vi "Init P2P stream.vi"(7 "single shot":bool, 8 "Trigger ource":T1, 9 "input impedance":u32(ring) caption="Input Impedance" items=["1 mega ohm"=0, "50 ohms"=2], 10 "SCOPE Resource":refnum<k15>="Dev1" caption="NI-Scope Resource", 11 "FPGA VI Reference":T3) -> (0 "error out":errorcluster, 2 "P2P params":T2={"instrument handle"="", "stream session"=refnum, "scale"={"offset"=0.0, "gain"=0.0, "reserved 1"=0.0, "reserved 2"=0.0}, "actual sample rate"=10000000.0, "Trigger"=enum."PFI 0", "SCOPE Resource"="Dev1", "input impedance"=0} {"input impedance" items=["1 mega ohm"=0, "50 ohms"=2]; "actual sample rate" format="%.2p"}, 3 "FPGA VI Reference out":T3)   [LabVIEW 2013]
uses:
  Config/5160FPGAref.ctl
  P2P params.ctl
  trigger_source.ctl
  <instrlib>/niScope/Controls/niScope vertical coupling.ctl
  <instrlib>/niScope/Controls/niScope trigger slope.ctl
  <instrlib>/niScope/Controls/niScope trigger source digital.ctl
  <instrlib>/niScope/Acquire/niScope Get Scaling Coefficients.vi
  <vilib>/FPGAPlugInAG/Dynamic/niLvFpga_P2PGetEndpoint_Dynamic.vi
  <instrlib>/niScope/Configure/Trigger/niScope Configure Trigger Software.vi
  <instrlib>/niScope/Configure/Trigger/niScope Configure Trigger Digital.vi
  <vilib>/rvi/interface/nirviMethod/nirviMethod.xnode
  <vilib>/rvi/errors/niLvFpgaMergeErrorWithErrorCode.vi
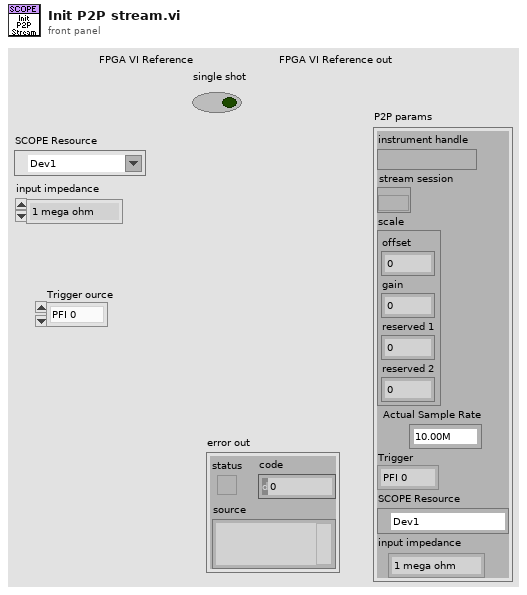
[diagram p1: front panel]
types:
  T1 = typedef "trigger_source.ctl" = enum16{"PFI 0", "PFI 1", "Software"}
  T2 = typedef "P2P params.ctl" = cluster{"instrument handle":refnum<k15>, "stream session":refnum<k20>, "scale":cluster{"offset":dbl, "gain":dbl, "reserved 1":dbl, "reserved 2":dbl}, "actual sample rate":dbl, "Trigger":T1, "SCOPE Resource":refnum<k15>, "input impedance":u32}
  T3 = typedef "5160FPGAref.ctl" = refnum<k20>
  T4 = typedef "niScope vertical coupling.ctl" = i32
  T5 = cluster{"offset":dbl, "gain":dbl, "reserved 1":dbl, "reserved 2":dbl}[]
  T6 = cluster{"coefficient info[0]":cluster{"offset":dbl, "gain":dbl, "reserved 1":dbl, "reserved 2":dbl}, "coefficient info[1]":cluster{"offset":dbl, "gain":dbl, "reserved 1":dbl, "reserved 2":dbl}, "coefficient info[2]":cluster{"offset":dbl, "gain":dbl, "reserved 1":dbl, "reserved 2":dbl}, "coefficient info[3]":cluster{"offset":dbl, "gain":dbl, "reserved 1":dbl, "reserved 2":dbl}, "coefficient info[4]":cluster{"offset":dbl, "gain":dbl, "reserved 1":dbl, "reserved 2":dbl}, "coefficient info[5]":cluster{"offset":dbl, "gain":dbl, "reserved 1":dbl, "reserved 2":dbl}, "coefficient info[6]":cluster{"offset":dbl, "gain":dbl, "reserved 1":dbl, "reserved 2":dbl}, "coefficient info[7]":cluster{"offset":dbl, "gain":dbl, "reserved 1":dbl, "reserved 2":dbl}, "coefficient info[8]":cluster{"offset":dbl, "gain":dbl, "reserved 1":dbl, "reserved 2":dbl}}
  T7 = typedef "niScope trigger source digital.ctl" = string
  T8 = typedef "niScope trigger slope.ctl" = i32
  T9 = cluster{"offset":dbl, "gain":dbl, "reserved 1":dbl, "reserved 2":dbl}
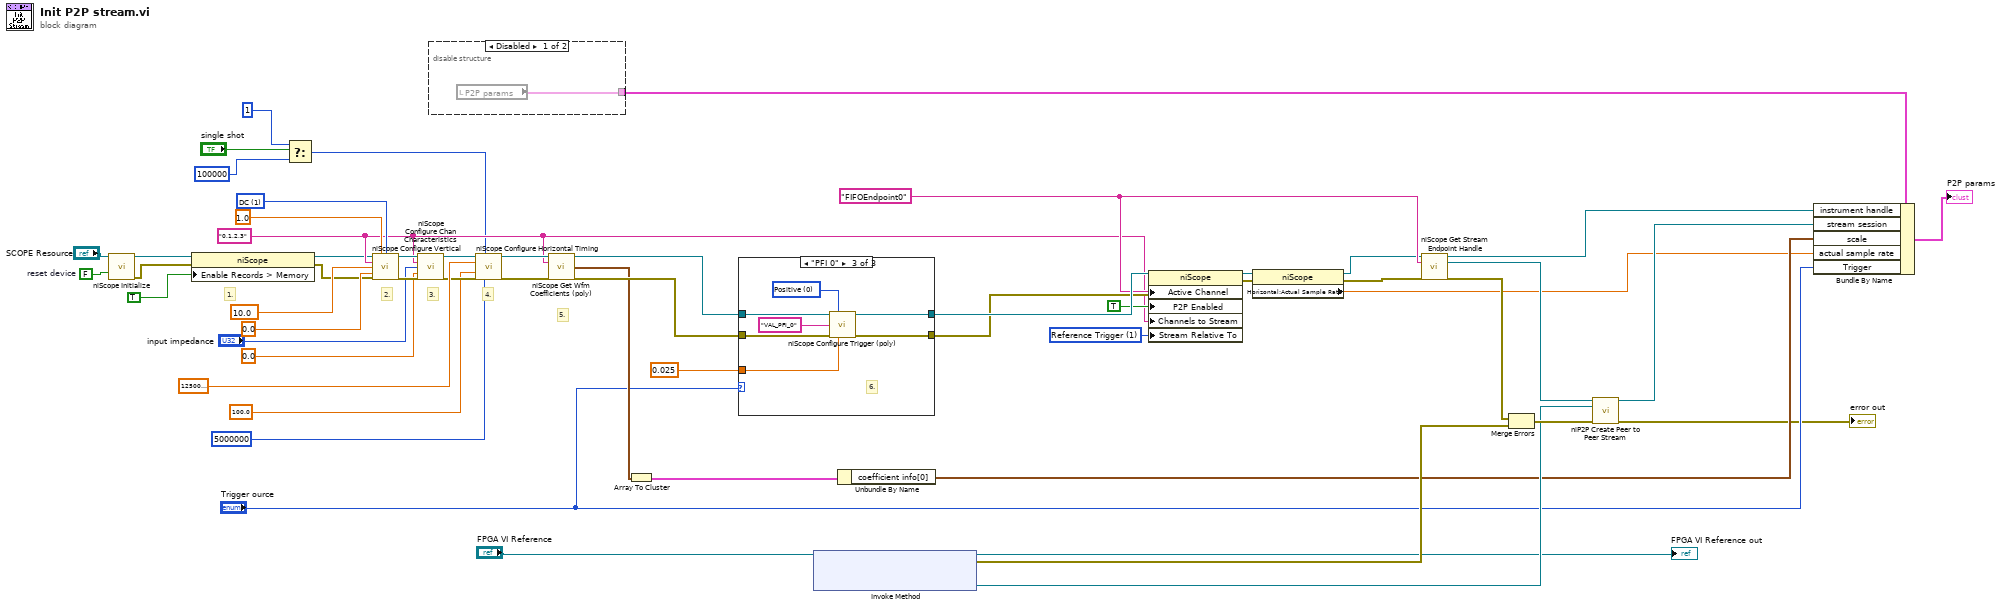
[diagram p0: block diagram]
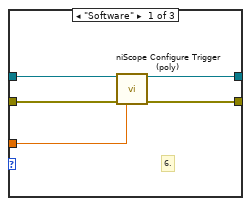
[diagram p2: hidden frame]
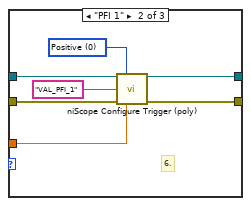
[diagram p3: hidden frame]
diagram:
  w15 = 1 items=["Start Trigger", "Reference Trigger", "Sync Trigger"] ("Peer-to-Peer:Stream Relative To")
  w44 = T4 1 items=["AC", "DC", "Ground"] ("vertical coupling")
  w34 = "0,1,2,3" ("channel name")
  w40 = "FIFOEndpoint0" ("Active Channel")
  w56 = FALSE  # reset device
  # "5."
  # "4."
  # "3."
  # "2."
  # "1."
  n1 = call <instrlib>:"niScope Initialize.vi"("resource name"="SCOPE Resource", "reset device"=w56) -> ("instrument handle"=w11:refnum<k15>, "error out"=w9:errorcluster)  [unwired: 12 in]
  n2 = property class="niScope"(reference=w11, error in=w9, "Enable Records > Memory"=TRUE ("Horizontal:Enable Records > Memory")) -> (reference out=w10:refnum<k15>, error out=w8:errorcluster)
  n3 = Select(t=1, s="single shot", f=100000 ("number of records")) -> (s? t:f=w2:i32)
  n4 = call <instrlib>:"niScope Configure Vertical.vi"("instrument handle"=w10, "probe attenuation"=1.0, "vertical coupling"=w44, "channels"=w34, "vertical range"=10.0, "vertical offset"=0.0, "error in"=w8) -> ("instrument handle out"=w52:refnum<k15>, "error out"=w51:errorcluster)  [unwired: 7 in]
  n5 = call <instrlib>:"niScope Configure Chan Characteristics.vi"("instrument handle"=w52, "channels"=w34, "input impedance"="input impedance", "maximum input frequency"=0.0, "error in"=w51) -> ("instrument handle out"=w49:refnum<k15>, "error out"=w50:errorcluster)  [unwired: 9 in]
  n6 = disable-structure shown="Disabled" {
    disable-tunnel: [w57 _] -> w21
    frame Disabled {
      n7 = local read "P2P params"() -> (w57:T2)
    }
    frame Enabled {
    }
  }
  n8 = call <instrlib>:"niScope Configure Horizontal Timing.vi"("instrument handle"=w49, "number of records"=w2, "min sample rate"=1250000000.0, "reference position"=100.0, "error in"=w50, "min record length"=5000000) -> ("instrument handle out"=w38:refnum<k15>, "error out"=w37:errorcluster)  [unwired: 8 in]
  n9 = call-poly <instrlib>:"niScope Get Wfm Coefficients (poly).vi"("instrument handle"=w38, "channels"=w34, "error in"=w37) -> ("instrument handle out"=w36:refnum<k15>, "coefficient info"=w33:T5, "error out"=w35:errorcluster)  [unwired: 10 in]
  n10 = Array To Cluster(array=w33) -> (cluster=w32:T6)
  n11 = case shown="\"PFI 0\"" "Trigger ource" {
    tunnel: [w62 w69 w76] -> w43
    tunnel: [w61 w68 w75] -> w42
    tunnel: w36 -> [w60 w67 w74]
    tunnel: w35 -> [w59 w66 w73]
    tunnel: 0.025 ("trigger holdoff") -> [w58 w65 w72]
    frame "Software" {
      # "6."
      n12 = call-poly <instrlib>:"niScope Configure Trigger (poly).vi"("instrument handle"=w60, "error in"=w59, "trigger holdoff"=w58) -> ("instrument handle out"=w62:refnum<k15>, "error out"=w61:errorcluster)  [unwired: 11 in]
    }
    frame "PFI 1" {
      w64 = T8 0 items=["Positive", "Negative"] ("trigger slope")
      # "6."
      n13 = call-poly <instrlib>:"niScope Configure Trigger (poly).vi"("instrument handle"=w67, "trigger slope"=w64, "trigger source"=T7 "VAL_PFI_1", "error in"=w66, "trigger holdoff"=w65) -> ("instrument handle out"=w69:refnum<k15>, "error out"=w68:errorcluster)  [unwired: 9 in]
    }
    frame "PFI 0" {
      w71 = T8 0 items=["Positive", "Negative"] ("trigger slope")
      # "6."
      n14 = call-poly <instrlib>:"niScope Configure Trigger (poly).vi"("instrument handle"=w74, "trigger slope"=w71, "trigger source"=T7 "VAL_PFI_0", "error in"=w73, "trigger holdoff"=w72) -> ("instrument handle out"=w76:refnum<k15>, "error out"=w75:errorcluster)  [unwired: 9 in]
    }
  }
  n15 = xnode "Invoke Method"("FPGA VI Reference In"="FPGA VI Reference") -> ("FPGA VI Reference Out"=→"FPGA VI Reference out":T3, "error out"=w23:errorcluster, "Reader"=w24:refnum<k20>)  [unwired: 1 in]
  n16 = Unbundle By Name(w32) -> ("coefficient info[0]"=w18:T9)
  n17 = property class="niScope"(reference=w43, error in=w42, "Active Channel"=w40, "P2P Enabled"=TRUE ("Peer-to-Peer:P2P Enabled"), "Channels to Stream"=w34, "Stream Relative To"=w15) -> (reference out=w29:refnum<k15>, error out=w28:errorcluster)
  n18 = property class="niScope"(reference=w29, error in=w28) -> (reference out=w26:refnum<k15>, error out=w27:errorcluster, "Horizontal:Actual Sample Rate"=w17:dbl)
  n19 = call <instrlib>:"niScope Get Stream Endpoint Handle.vi"("instrument handle"=w26, "stream endpoint"=w40, "error in"=w27) -> ("instrument handle out"=w7:refnum<k15>, "writer handle"=w39:refnum<k20>, "error out"=w30:errorcluster)  [unwired: 10 in]
  n20 = Merge Errors(w30, w23) -> (w31:errorcluster)
  n21 = call <vilib>:"niP2P Create Peer to Peer Stream.vi"("writer"=w39, "reader"=w24, "error in (no error)"=w31) -> ("stream session"=w20:refnum<k20>, "error out"=→"error out":errorcluster)  [unwired: 11 in]
  n22 = Bundle By Name(cluster=w21, "instrument handle"=w7, "stream session"=w20, "scale"=w18, "actual sample rate"=w17, "Trigger"="Trigger ource") -> (→"P2P params":T2)
